vi "error.handler.vi"(8 "error in (no error)":errorcluster, 11 "manager_daemon in":refnum<class "manager_daemon.lvclass">) -> (0 "error out":errorcluster, 3 "manager_daemon out":refnum<class "manager_daemon.lvclass">, 4 "exit":bool)   [LabVIEW 2024, in "manager_daemon.lvclass"]
uses:
  manager_daemon.lvclass
  manager_daemon.lvclass/manager_daemon.ctl
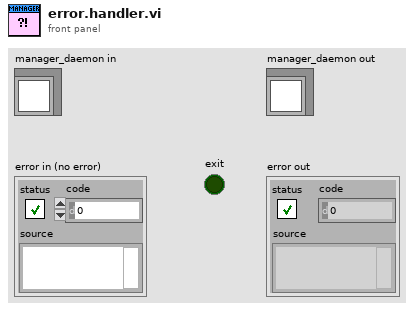
[diagram p1: front panel]
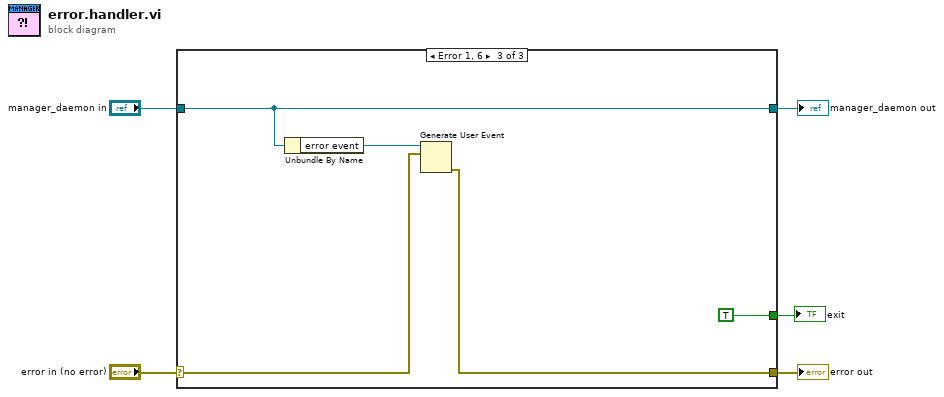
[diagram p0: block diagram]
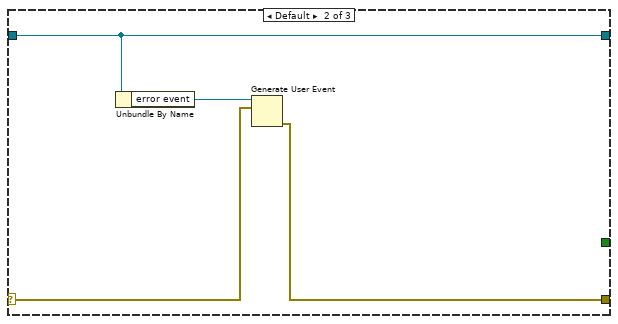
[diagram p3: hidden frame]
diagram:
  n1 = case shown="Error 1, 6" "error in (no error)" {
    selector: "error in (no error)" -> [w6 w9 w13]
    tunnel: [w6 w8 w12] -> w4
    tunnel: [w7 w11 w14] -> w2
    tunnel: "manager_daemon in" -> [w7 w11 w14]
    tunnel: [_ _ TRUE] -> w1
    frame No Error {
    }
    frame Default {
      n2 = Unbundle By Name(w11) -> ("error event"=w10:refnum<user-event>)
      n3 = Generate User Event(user event=w10, event data cluster=w9) -> (error out=w8:errorcluster)  [unwired: 2 in, 1 out]
    }
    frame Error {
      n4 = Unbundle By Name(w14) -> ("error event"=w15:refnum<user-event>)
      n5 = Generate User Event(user event=w15, event data cluster=w13) -> (error out=w12:errorcluster)  [unwired: 2 in, 1 out]
    }
  }
  "error out" <- w4
  "manager_daemon out" <- w2
  "exit" <- w1
